vi "autocenter.vi"() -> ()   [LabVIEW 2012, in "Mecanum Drive.lvrbt"]
uses:
  Mecanum Drive.lvrbt
  SubVIs/State_Typ.ctl
  <vilib>/NXT/HiTechnic/HiTechnic Controls/HiTechnic Port.ctl
  <vilib>/NXT/Block Support/NXT_InputPort.ctl
  SubVIs/auto_drive_TYP.ctl
  <vilib>/NXT/Hardware/Plugins/Tetrix DC Motor/TetrixDCMotorAddress.ctl
  <vilib>/NXT/Dual Mode Library/Display/drawNumber.vi
  <vilib>/NXT/NXTIO Xnodes/NXTIONodeSubVIs/TETRIX IO Check Battery.vi
  <vilib>/NXT/Dual Mode Library/Waits/Wait_Num(msec).vi
  <vilib>/NXT/NXTIO Xnodes/NXTIONodeSubVIs/TETRIX IO Reset Encoders.vi
  <vilib>/NXT/NXTIO Xnodes/NXTIONodeSubVIs/TETRIX IO Motor Status.vi
  <vilib>/NXT/NXTIO Xnodes/NXTIONodeSubVIs/TETRIX IO Stop DC Motors.vi
  <vilib>/NXT/Dual Mode Library/Sound/Tone.vi
  <vilib>/NXT/Dual Mode Library/Waits/Wait_Num.vi
  <vilib>/NXT/Subs/LVHSConnector.ctl
  <vilib>/NXT/NXTIO Xnodes/AddressXNode/NXTIOAddress.xnode
  <vilib>/NXT/NXTIO Xnodes/NXTIOXNode/NXTIO.xnode
  <vilib>/NXT/LegoClasses/BrickReference/BrickReference.lvclass
panel:
  out "Enabled":bool
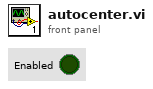
[diagram p1: front panel]
types:
  T1 = typedef "auto_drive_TYP.ctl" = cluster{"Left X":i8, "Left Y":i8, "Right X":i8, "Power (100)":i8, "Wait (ms)":u32, "Enc/Deg Target":i32, "Move Type":enum16{"Relative Degrees", "Wait", "Encoder"}}
  T2 = typedef "State_Typ.ctl" = enum16{"Stop", "Check for Position 3", "Check for Position 2", "Move", "Reset Enc", "Read Enc"}
  T3 = typedef "HiTechnic Port.ctl" = cluster{"Port":T4, "MUX Port":u8}
  T4 = typedef "NXT_InputPort.ctl" = u32
  T5 = typedef "TetrixDCMotorAddress.ctl" = i32
  T6 = typedef "LVHSConnector.ctl" = refnum<class "BrickReference.lvclass">
  T7 = cluster{"TetrixDCMotor":T5, "TetrixDCMotor 2":T5}
  T8 = cluster{"Direction (0-9)":i16, "Signal Strength (Array)":u8[]}
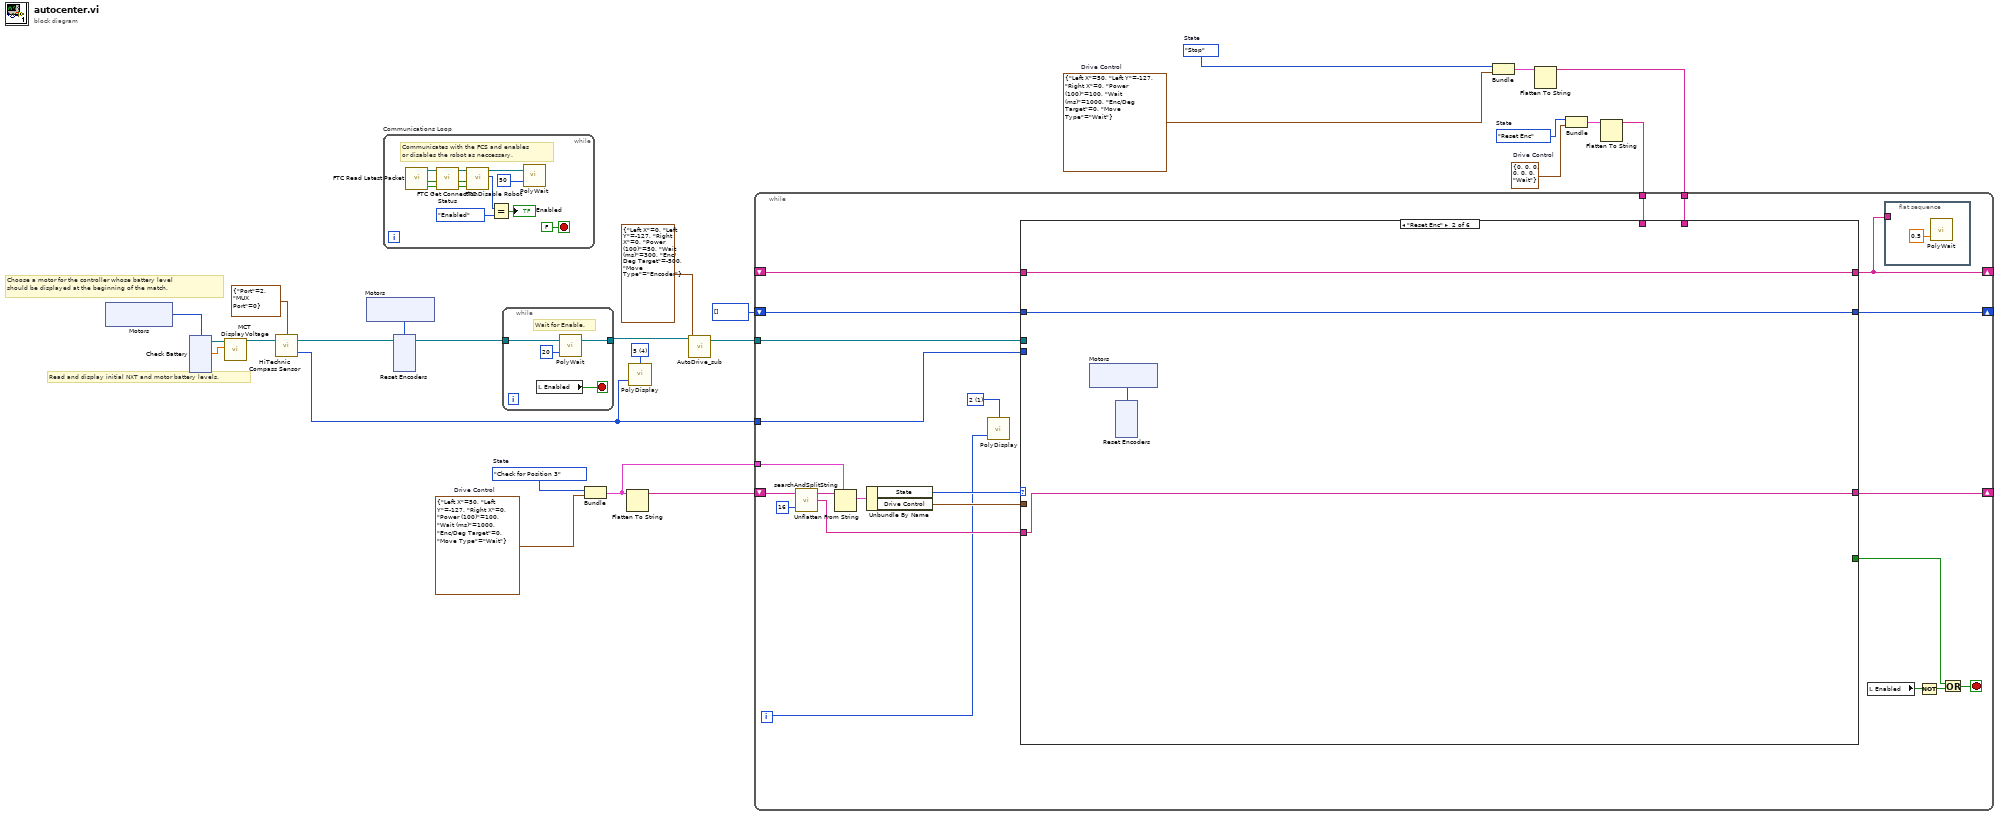
[diagram p0: block diagram]
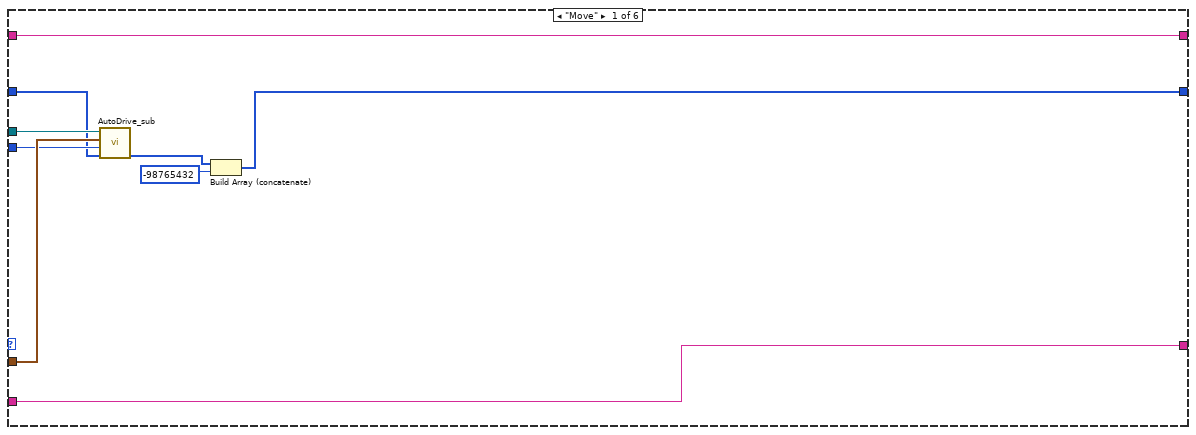
[diagram p2: hidden frame]
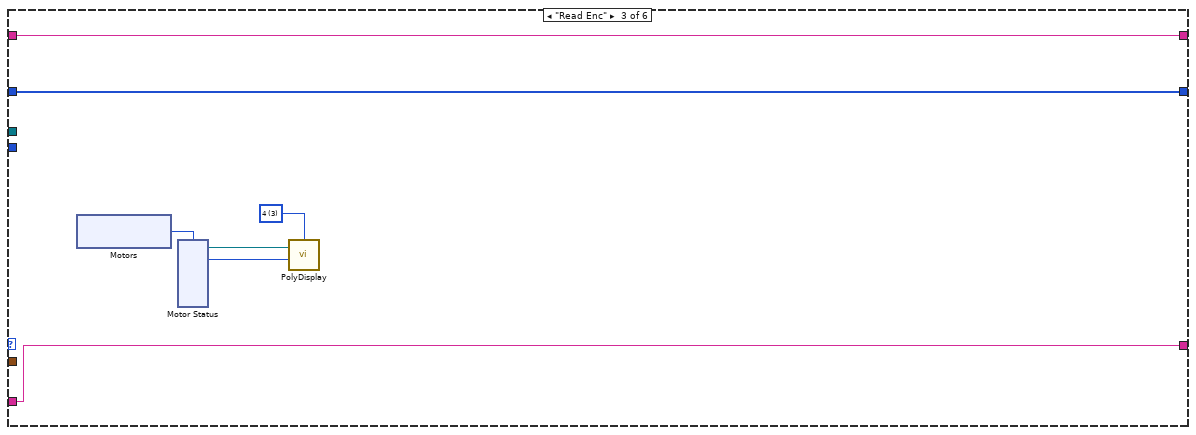
[diagram p3: hidden frame]
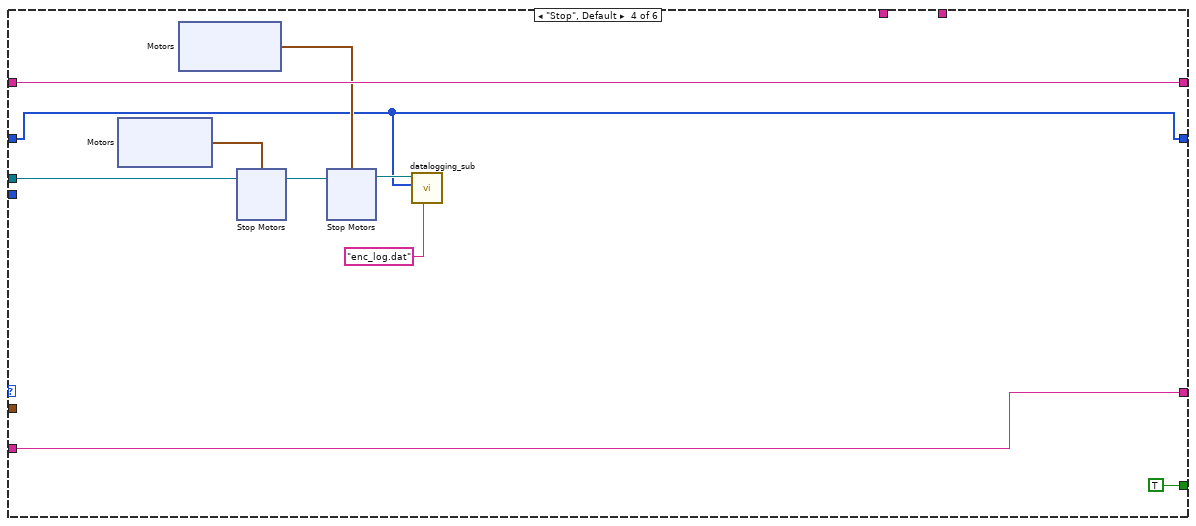
[diagram p4: hidden frame]
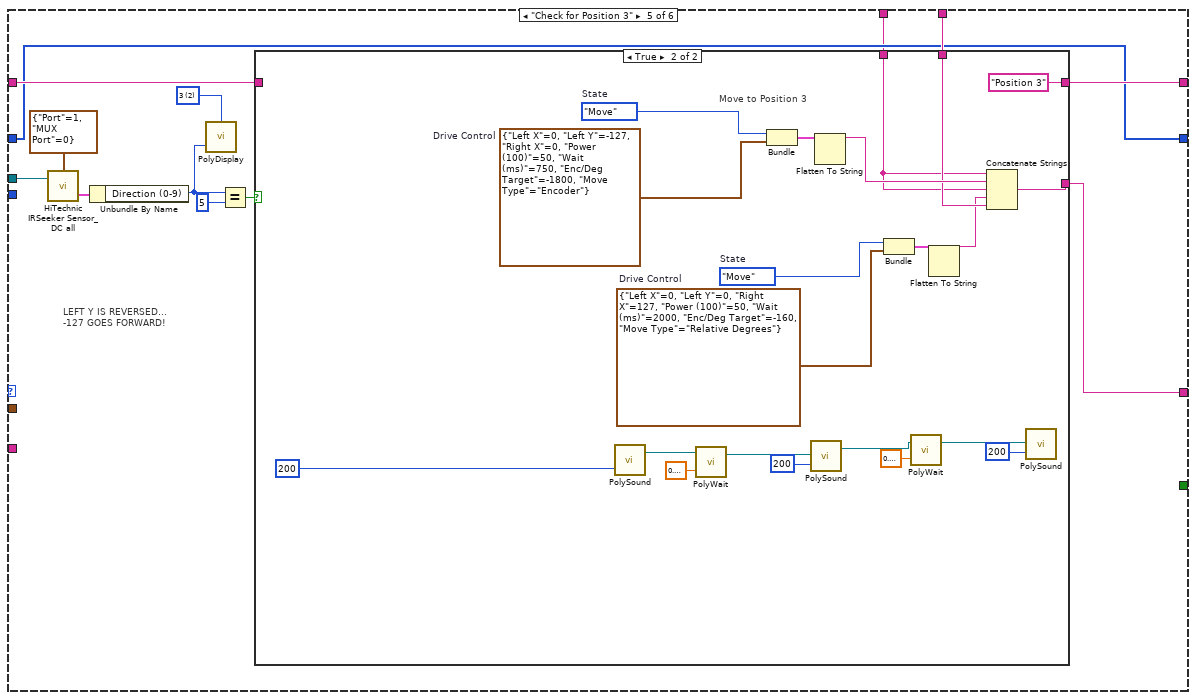
[diagram p5: hidden frame]
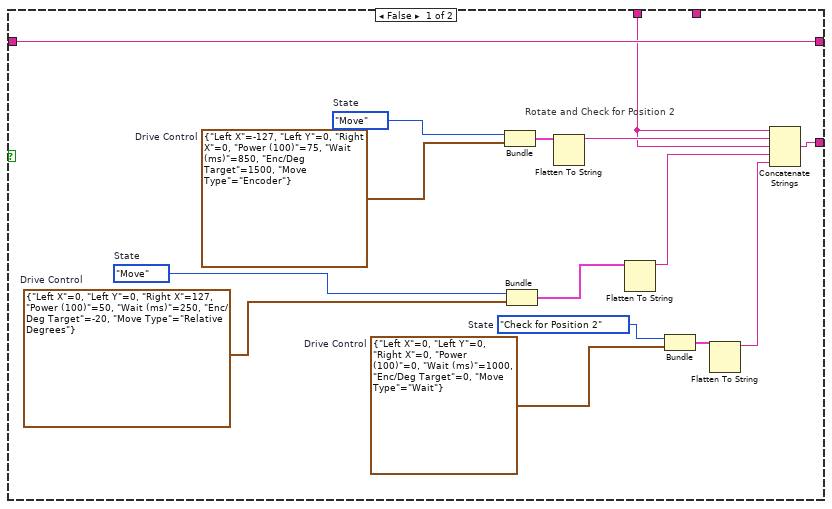
[diagram p6: hidden frame]
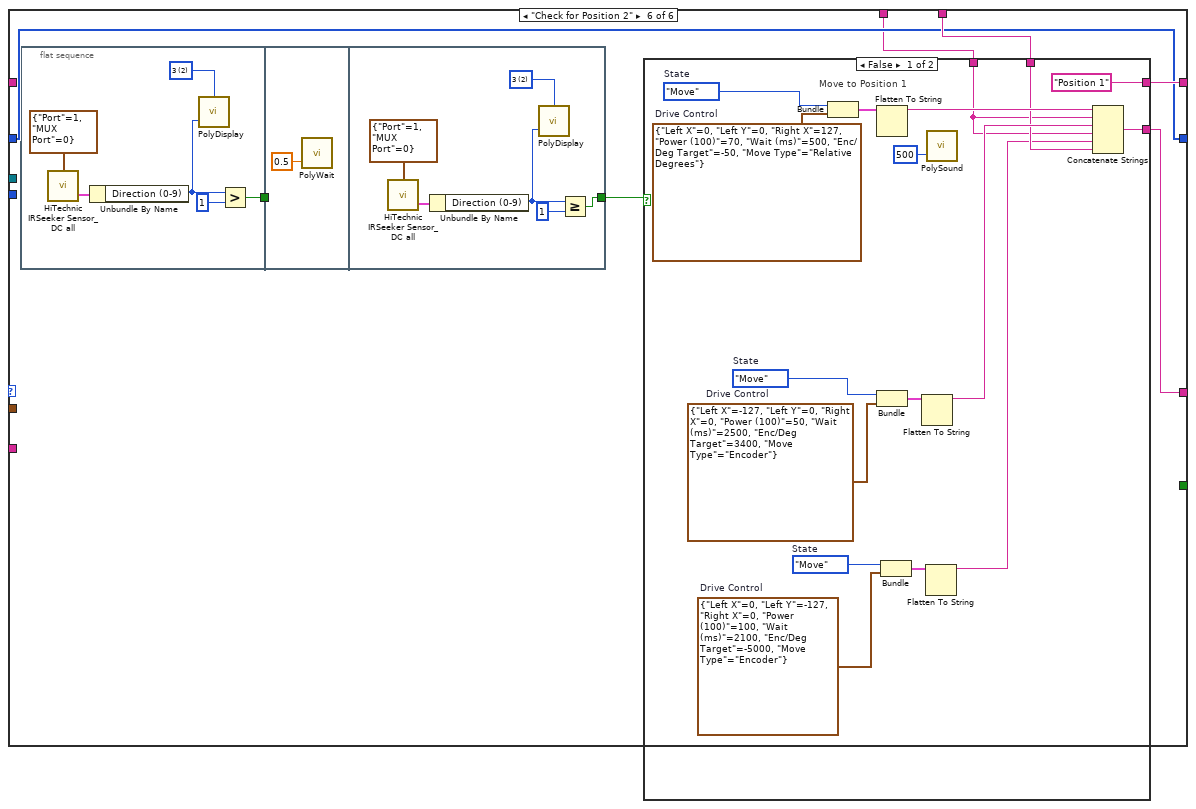
[diagram p7: hidden frame]
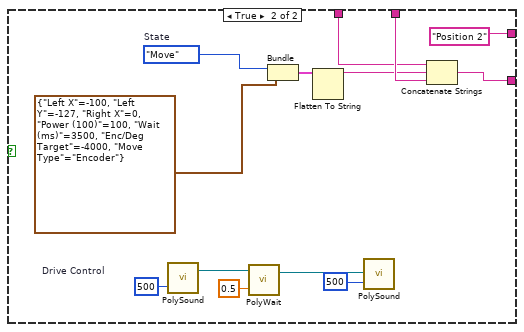
[diagram p8: hidden frame]
diagram:
  w4 = T1 {"Left X"=0, "Left Y"=0, "Right X"=0, "Power (100)"=0, "Wait (ms)"=0, "Enc/Deg Target"=0, "Move Type"=enum."Wait"}  # Drive Control
  w6 = State_Typ."Reset Enc"  # State
  w26 = T1 {"Left X"=50, "Left Y"=-127, "Right X"=0, "Power (100)"=100, "Wait (ms)"=1000, "Enc/Deg Target"=0, "Move Type"=enum."Wait"}  # Drive Control
  w13 = T1 {"Left X"=50, "Left Y"=-127, "Right X"=0, "Power (100)"=100, "Wait (ms)"=1000, "Enc/Deg Target"=0, "Move Type"=enum."Wait"}  # Drive Control
  w14 = State_Typ."Stop"  # State
  w17 = i16 4 items=["1", "2", "3", "4", "5", "6", "7", "8", "9", "10", "11", "12"] ("Line")
  w25 = State_Typ."Check for Position 3"  # State
  # "Read and display initial NXT and motor battery levels."
  # "Choose a motor for the controller whose battery level \nshould be displayed at the beginning of the match."
  n1 = xnode "Motors"() -> ("Motor"=w22:T5)
  n2 = xnode "Check Battery"("Motors"=w22) -> ("Voltage 1"=w23:sgl, "NXT/EV3"=w24:T6)  [unwired: 1 in]
  n3 = call <vilib>:"MCT DisplayVoltage.vi"("Motor Voltage"=w23, "NXT"=w24) -> ("NXT"=w18:T6)  [unwired: 9 in]
  n4 = call <vilib>:"HiTechnic Compass Sensor.vi"("NXT/EV3"=w18, "Port/MUX"=T3 {"Port"=2, "MUX Port"=0}) -> ("Heading (degrees)"=w16:i16, "NXT/EV3"=w2:T6)  [unwired: 1 in]
  n5 = xnode "Motors"() -> ("Motor"=w3:T5)
  n6 = while "Communications Loop" {
    stop <- FALSE stop-if-true
    # "Communicates with the FCS and enables \nor disables the robot as neccessary."
    n7 = call <vilib>:"FTC Read Latest Packet.vi"() -> ("Packet Received?"=w36:bool, "Stopped?"=w35:bool, "NXT"=w38:T6)  [unwired: 6 in, 3 out]
    n8 = call <vilib>:"FTC Get Connection Status.vi"("Packet Received?"=w36, "Stopped?"=w35, "NXT"=w38) -> ("Online?"=w27:bool, "Stopped?"=w28:bool, "NXT"=w37:T6)  [unwired: 5 in]
    n9 = call <vilib>:"FTC Disable Robot.vi"("Online?"=w27, "Stopped?"=w28, "NXT"=w37) -> ("Enabled?"=w31:enum16{"Disabled", "Enabled"}, "NXT"=w33:T6)  [unwired: 3 in]
    n10 = Equal?(x=w31, y=enum16{"Disabled", "Enabled"}."Enabled") -> (x = y?=→"Enabled":bool)
    n11 = call-poly <vilib>:"PolyWait.vi"("Time (100 msec)"=u32 50 ("Time (msec)"), "NXT/EV3"=w33) -> ()  [unwired: 2 in, 1 out]
  }
  n12 = xnode "Reset Encoders"("Motors"=w3, "NXT/EV3"=w2) -> ("NXT/EV3"=w1:T6)
  n13 = while {
    tunnel: [w40] -> w10
    tunnel: w1 -> [w39]
    stop <- w41 stop-if-true
    # "Wait for Enable."
    n14 = local read "Enabled"() -> (w41:bool)
    n15 = call-poly <vilib>:"PolyWait.vi"("Time (100 msec)"=u32 20 ("Time (msec)"), "NXT/EV3"=w39) -> ("NXT/EV3"=w40:T6)  [unwired: 2 in]
  }
  n16 = Bundle("State"=w25, "Drive Control"=w26) -> (w21:cluster{"State":T2, "Drive Control":T1})  [unwired: 1 in]
  n17 = Flatten To String(anything=w21) -> (data string=w20:string)  [unwired: 3 in, 2 out]
  n18 = call-poly <vilib>:"PolyDisplay.vi"("number"=w16, "Line"=w17) -> ()  [unwired: 2 in, 1 out]
  n19 = call "AutoDrive_sub.vi"("Drive Control"=T1 {"Left X"=0, "Left Y"=-127, "Right X"=0, "Power (100)"=50, "Wait (ms)"=300, "Enc/Deg Target"=-500, "Move Type"=enum."Encoder"}, "NXT/EV3"=w10) -> ("NXT/EV3 out"=w11:T6)  [unwired: 8 in, 1 out]
  n20 = Bundle("State"=w14, "Drive Control"=w13) -> (w15:cluster{"State":T2, "Drive Control":T1})  [unwired: 1 in]
  n21 = Flatten To String(anything=w15) -> (data string=w12:string)  [unwired: 3 in, 2 out]
  n22 = Bundle("State"=w6, "Drive Control"=w4) -> (w7:cluster{"State":T2, "Drive Control":T1})  [unwired: 1 in]
  n23 = Flatten To String(anything=w7) -> (data string=w5:string)  [unwired: 3 in, 2 out]
  n24 = while {
    tunnel: w11 -> [w65]
    shift-right: [w56] -> _
    shift-left: w20 -> [w54]
    tunnel: w21 -> [w57]
    shift-right: [w47] -> _
    shift-left: _ -> [w55]
    tunnel: w12 -> [w52]
    tunnel: w16 -> [w46]
    shift-right: [w45] -> _
    shift-left: i32[] [] -> [w44]
    tunnel: w5 -> [w43]
    i -> [w48]
    stop <- w64 stop-if-true
    w49 = i16 1 items=["1", "2", "3", "4", "5", "6", "7", "8", "9", "10", "11", "12"] ("Line")
    n25 = call <vilib>:"searchAndSplitString.vi"("offset (0)"=16 ("length (rest)"), "string"=w54) -> ("match + rest of string"=w53:string, "substring before match"=w59:string)  [unwired: 1 in, 1 out]
    n26 = Unflatten From String(type=w57, binary string=w59) -> (value=w58:cluster{"State":T2, "Drive Control":T1})  [unwired: 3 in, 2 out]
    n27 = Unbundle By Name(w58) -> ("State"=w50:T2, "Drive Control"=w60:T1)
    n28 = call-poly <vilib>:"PolyDisplay.vi"("number"=w48, "Line"=w49) -> ()  [unwired: 2 in, 1 out]
    n29 = case shown="\"Reset Enc\"" w50 {
      tunnel: w65 -> [w75 _ _ w110 w133 _]
      tunnel: [_ _ _ TRUE _ _] -> w63
      tunnel: w60 -> [w74 _ _ _ _ _]
      tunnel: w53 -> [w73 w79 w91 w108 _ _]
      tunnel: [w73 w79 w91 w108 w129 w175] -> w56
      tunnel: [w72 w78 w90 w107 w132 w177] -> w47
      tunnel: w55 -> [w72 w78 w90 w107 w131 _]
      tunnel: w52 -> [_ _ _ _ w130 w176]
      tunnel: w46 -> [w71 _ _ _ _ _]
      tunnel: [w70 w76 w85 w102 w124 w173] -> w45
      tunnel: w44 -> [w68 w76 w85 w102 w124 w173]
      tunnel: w43 -> [_ _ _ _ w123 w172]
      frame "Move" {
        n30 = call "AutoDrive_sub.vi"("EncoderVals"=w68, "Target Heading (Degrees)"=w71, "Drive Control"=w74, "NXT/EV3"=w75) -> ("EncoderVals"=w67:i32[])  [unwired: 6 in, 1 out]
        n31 = Build Array (concatenate)(w67, -98765432 ("new element/subarray")) -> (w70:i32[])
      }
      frame "Reset Enc" {
        n32 = xnode "Motors"() -> ("Motor"=w77:T5)
        n33 = xnode "Reset Encoders"("Motors"=w77) -> ()  [unwired: 1 in, 1 out]
      }
      frame "Read Enc" {
        w87 = i16 3 items=["1", "2", "3", "4", "5", "6", "7", "8", "9", "10", "11", "12"] ("Line")
        n34 = xnode "Motors"() -> ("Motor"=w89:T5)
        n35 = xnode "Motor Status"("Motors"=w89) -> ("Position 1"=w88:i32, "NXT/EV3"=w86:T6)  [unwired: 1 in, 1 out]
        n36 = call-poly <vilib>:"PolyDisplay.vi"("number"=w88, "NXT/EV3"=w86, "Line"=w87) -> ()  [unwired: 1 in, 1 out]
      }
      frame "Stop", Default {
        n37 = xnode "Motors"() -> ("Motor"=w106:cluster{"TetrixDCMotor":T5, "TetrixDCMotor":T5})
        n38 = xnode "Motors"() -> ("Motor"=w105:cluster{"TetrixDCMotor":T5, "TetrixDCMotor":T5})
        n39 = xnode "Stop Motors"("Motors"=w106, "NXT/EV3"=w110) -> ("NXT/EV3"=w104:T6)
        n40 = xnode "Stop Motors"("Motors"=w105, "NXT/EV3"=w104) -> ("NXT/EV3"=w103:T6)
        n41 = call "datalogging_sub.vi"("Filename"="enc_log.dat", "Encoder Vals"=w102, "NXT/EV3 In"=w103) -> ()  [unwired: 8 in, 1 out]
      }
      frame "Check for Position 3" {
        w126 = i16 2 items=["1", "2", "3", "4", "5", "6", "7", "8", "9", "10", "11", "12"] ("Line")
        # "LEFT Y IS REVERSED...\n-127 GOES FORWARD!"
        n42 = call <vilib>:"HiTechnic IRSeeker Sensor_DC all.vi"("NXT/EV3"=w133, "Port/MUX"=T3 {"Port"=1, "MUX Port"=0}) -> ("All Info"=w135:T8)  [unwired: 1 in, 1 out]
        n43 = Unbundle By Name(w135) -> ("Direction (0-9)"=w127:i16)
        n44 = call-poly <vilib>:"PolyDisplay.vi"("number"=w127, "Line"=w126) -> ()  [unwired: 2 in, 1 out]
        n45 = Equal?(x=w127, y=i16 5) -> (x = y?=w125:bool)
        n46 = case shown="True" w125 {
          tunnel: [w145 w164] -> w129
          tunnel: [w144 "Position 3"] -> w132
          tunnel: w131 -> [w144 _]
          tunnel: w130 -> [_ w162]
          tunnel: w123 -> [w136 w151]
          frame False {
            w140 = T1 {"Left X"=0, "Left Y"=0, "Right X"=127, "Power (100)"=50, "Wait (ms)"=250, "Enc/Deg Target"=-20, "Move Type"=enum."Relative Degrees"}  # Drive Control
            w141 = State_Typ."Move"  # State
            w149 = T1 {"Left X"=0, "Left Y"=0, "Right X"=0, "Power (100)"=0, "Wait (ms)"=1000, "Enc/Deg Target"=0, "Move Type"=enum."Wait"}  # Drive Control
            w150 = State_Typ."Check for Position 2"  # State
            w143 = T1 {"Left X"=-127, "Left Y"=0, "Right X"=0, "Power (100)"=75, "Wait (ms)"=850, "Enc/Deg Target"=1500, "Move Type"=enum."Encoder"}  # Drive Control
            w146 = State_Typ."Move"  # State
            # "Rotate and Check for Position 2"
            n47 = Bundle("State"=w146, "Drive Control"=w143) -> (w147:cluster{"State":T2, "Drive Control":T1})  [unwired: 1 in]
            n48 = Bundle("State"=w141, "Drive Control"=w140) -> (w142:cluster{"State":T2, "Drive Control":T1})  [unwired: 1 in]
            n49 = Flatten To String(anything=w147) -> (data string=w137:string)  [unwired: 3 in, 2 out]
            n50 = Flatten To String(anything=w142) -> (data string=w139:string)  [unwired: 3 in, 2 out]
            n51 = Bundle("State"=w150, "Drive Control"=w149) -> (w148:cluster{"State":T2, "Drive Control":T1})  [unwired: 1 in]
            n52 = Flatten To String(anything=w148) -> (data string=w138:string)  [unwired: 3 in, 2 out]
            n53 = Concatenate Strings(w136, w137, w136, w139, w138) -> (w145:string)
          }
          frame True {
            w168 = T1 {"Left X"=0, "Left Y"=0, "Right X"=127, "Power (100)"=50, "Wait (ms)"=2000, "Enc/Deg Target"=-160, "Move Type"=enum."Relative Degrees"}  # Drive Control
            w169 = State_Typ."Move"  # State
            w171 = T1 {"Left X"=0, "Left Y"=-127, "Right X"=0, "Power (100)"=50, "Wait (ms)"=750, "Enc/Deg Target"=-1800, "Move Type"=enum."Encoder"}  # Drive Control
            w170 = State_Typ."Move"  # State
            # "Move to Position 3"
            n54 = call-poly <vilib>:"PolySound.vi"("Duration (500 ms)"=u16 200) -> ("NXT/EV3"=w158:T6)  [unwired: 3 in]
            n55 = call-poly <vilib>:"PolyWait.vi"("Time (1 sec)"=sgl 0.2, "NXT/EV3"=w158) -> ("NXT/EV3"=w157:T6)  [unwired: 2 in]
            n56 = Bundle("State"=w170, "Drive Control"=w171) -> (w167:cluster{"State":T2, "Drive Control":T1})  [unwired: 1 in]
            n57 = call-poly <vilib>:"PolySound.vi"("Duration (500 ms)"=u16 200, "NXT/EV3"=w157) -> ("NXT/EV3"=w154:T6)  [unwired: 2 in]
            n58 = Flatten To String(anything=w167) -> (data string=w165:string)  [unwired: 3 in, 2 out]
            n59 = Bundle("State"=w169, "Drive Control"=w168) -> (w166:cluster{"State":T2, "Drive Control":T1})  [unwired: 1 in]
            n60 = call-poly <vilib>:"PolyWait.vi"("Time (1 sec)"=sgl 0.2, "NXT/EV3"=w154) -> ("NXT/EV3"=w153:T6)  [unwired: 2 in]
            n61 = Flatten To String(anything=w166) -> (data string=w152:string)  [unwired: 3 in, 2 out]
            n62 = Concatenate Strings(w151, w165, w151, w152, w162) -> (w164:string)
            n63 = call-poly <vilib>:"PolySound.vi"("Duration (500 ms)"=u16 200, "NXT/EV3"=w153) -> ()  [unwired: 2 in, 1 out]
          }
        }
      }
      frame "Check for Position 2" {
        n64 = flat-sequence {
          tunnel: [w182] -> w174
          tunnel: w174 -> [_]
          tunnel: [w186] -> w178
          frame #0 {
            w179 = i16 2 items=["1", "2", "3", "4", "5", "6", "7", "8", "9", "10", "11", "12"] ("Line")
            n65 = call <vilib>:"HiTechnic IRSeeker Sensor_DC all.vi"("Port/MUX"=T3 {"Port"=1, "MUX Port"=0}) -> ("All Info"=w184:T8)  [unwired: 2 in, 1 out]
            n66 = Unbundle By Name(w184) -> ("Direction (0-9)"=w180:i16)
            n67 = call-poly <vilib>:"PolyDisplay.vi"("number"=w180, "Line"=w179) -> ()  [unwired: 2 in, 1 out]
            n68 = Greater?(x=w180, y=i16 1) -> (0:w182:bool)
          }
          frame #1 {
            n69 = call-poly <vilib>:"PolyWait.vi"("Time (1 sec)"=sgl 0.5) -> ()  [unwired: 3 in, 1 out]
          }
          frame #2 {
            w191 = i16 2 items=["1", "2", "3", "4", "5", "6", "7", "8", "9", "10", "11", "12"] ("Line")
            n70 = call <vilib>:"HiTechnic IRSeeker Sensor_DC all.vi"("Port/MUX"=T3 {"Port"=1, "MUX Port"=0}) -> ("All Info"=w187:T8)  [unwired: 2 in, 1 out]
            n71 = Unbundle By Name(w187) -> ("Direction (0-9)"=w190:i16)
            n72 = call-poly <vilib>:"PolyDisplay.vi"("number"=w190, "Line"=w191) -> ()  [unwired: 2 in, 1 out]
            n73 = Greater Or Equal?(x=w190, y=i16 1) -> (x >= y?=w186:bool)
          }
        }
        n74 = case shown="False" w178 {
          tunnel: [w205 w218] -> w175
          tunnel: ["Position 1" "Position 2"] -> w177
          tunnel: w176 -> [w197 w211]
          tunnel: w172 -> [w192 w209]
          frame False {
            w195 = T1 {"Left X"=0, "Left Y"=-127, "Right X"=0, "Power (100)"=100, "Wait (ms)"=2100, "Enc/Deg Target"=-5000, "Move Type"=enum."Encoder"}  # Drive Control
            w196 = State_Typ."Move"  # State
            w203 = T1 {"Left X"=-127, "Left Y"=0, "Right X"=0, "Power (100)"=50, "Wait (ms)"=2500, "Enc/Deg Target"=3400, "Move Type"=enum."Encoder"}  # Drive Control
            w204 = State_Typ."Move"  # State
            w207 = T1 {"Left X"=0, "Left Y"=0, "Right X"=127, "Power (100)"=70, "Wait (ms)"=500, "Enc/Deg Target"=-50, "Move Type"=enum."Relative Degrees"}  # Drive Control
            w208 = State_Typ."Move"  # State
            # "Move to Position 1"
            n75 = Bundle("State"=w208, "Drive Control"=w207) -> (w206:cluster{"State":T2, "Drive Control":T1})  [unwired: 1 in]
            n76 = Flatten To String(anything=w206) -> (data string=w199:string)  [unwired: 3 in, 2 out]
            n77 = Bundle("State"=w204, "Drive Control"=w203) -> (w202:cluster{"State":T2, "Drive Control":T1})  [unwired: 1 in]
            n78 = Bundle("State"=w196, "Drive Control"=w195) -> (w194:cluster{"State":T2, "Drive Control":T1})  [unwired: 1 in]
            n79 = Flatten To String(anything=w202) -> (data string=w201:string)  [unwired: 3 in, 2 out]
            n80 = Flatten To String(anything=w194) -> (data string=w193:string)  [unwired: 3 in, 2 out]
            n81 = call-poly <vilib>:"PolySound.vi"("Duration (500 ms)"=u16 500) -> ()  [unwired: 3 in, 1 out]
            n82 = Concatenate Strings(w199, w192, w201, w192, w193, w197) -> (w205:string)
          }
          frame True {
            w220 = T1 {"Left X"=-100, "Left Y"=-127, "Right X"=0, "Power (100)"=100, "Wait (ms)"=3500, "Enc/Deg Target"=-4000, "Move Type"=enum."Encoder"}  # Drive Control
            w219 = State_Typ."Move"  # State
            n83 = call-poly <vilib>:"PolySound.vi"("Duration (500 ms)"=u16 500) -> ("NXT/EV3"=w213:T6)  [unwired: 3 in]
            n84 = call-poly <vilib>:"PolyWait.vi"("Time (1 sec)"=sgl 0.5, "NXT/EV3"=w213) -> ("NXT/EV3"=w212:T6)  [unwired: 2 in]
            n85 = Bundle("State"=w219, "Drive Control"=w220) -> (w221:cluster{"State":T2, "Drive Control":T1})  [unwired: 1 in]
            n86 = Flatten To String(anything=w221) -> (data string=w210:string)  [unwired: 3 in, 2 out]
            n87 = call-poly <vilib>:"PolySound.vi"("Duration (500 ms)"=u16 500, "NXT/EV3"=w212) -> ()  [unwired: 2 in, 1 out]
            n88 = Concatenate Strings(w209, w210, w211) -> (w218:string)
          }
        }
      }
    }
    n89 = local read "Enabled"() -> (w62:bool)
    n90 = flat-sequence {
      tunnel: w47 -> [_]
      frame #0 {
        n91 = call-poly <vilib>:"PolyWait.vi"("Time (1 sec)"=sgl 0.5) -> ()  [unwired: 3 in, 1 out]
      }
    }
    n92 = Not(x=w62) -> (.not. x?=w51:bool)
    n93 = Or(x=w63, y=w51) -> (x .or. y?=w64:bool)
  }
